vi "cluster.vi"() -> ()   [LabVIEW 2021]
panel:
  out "Array 2":T1(array[cluster])
  in  "y":enum16{"O", "B-", "B+", "A-", "A+"}(ring)
  out "Application form":T2
  in  "Array":T1(array[cluster])
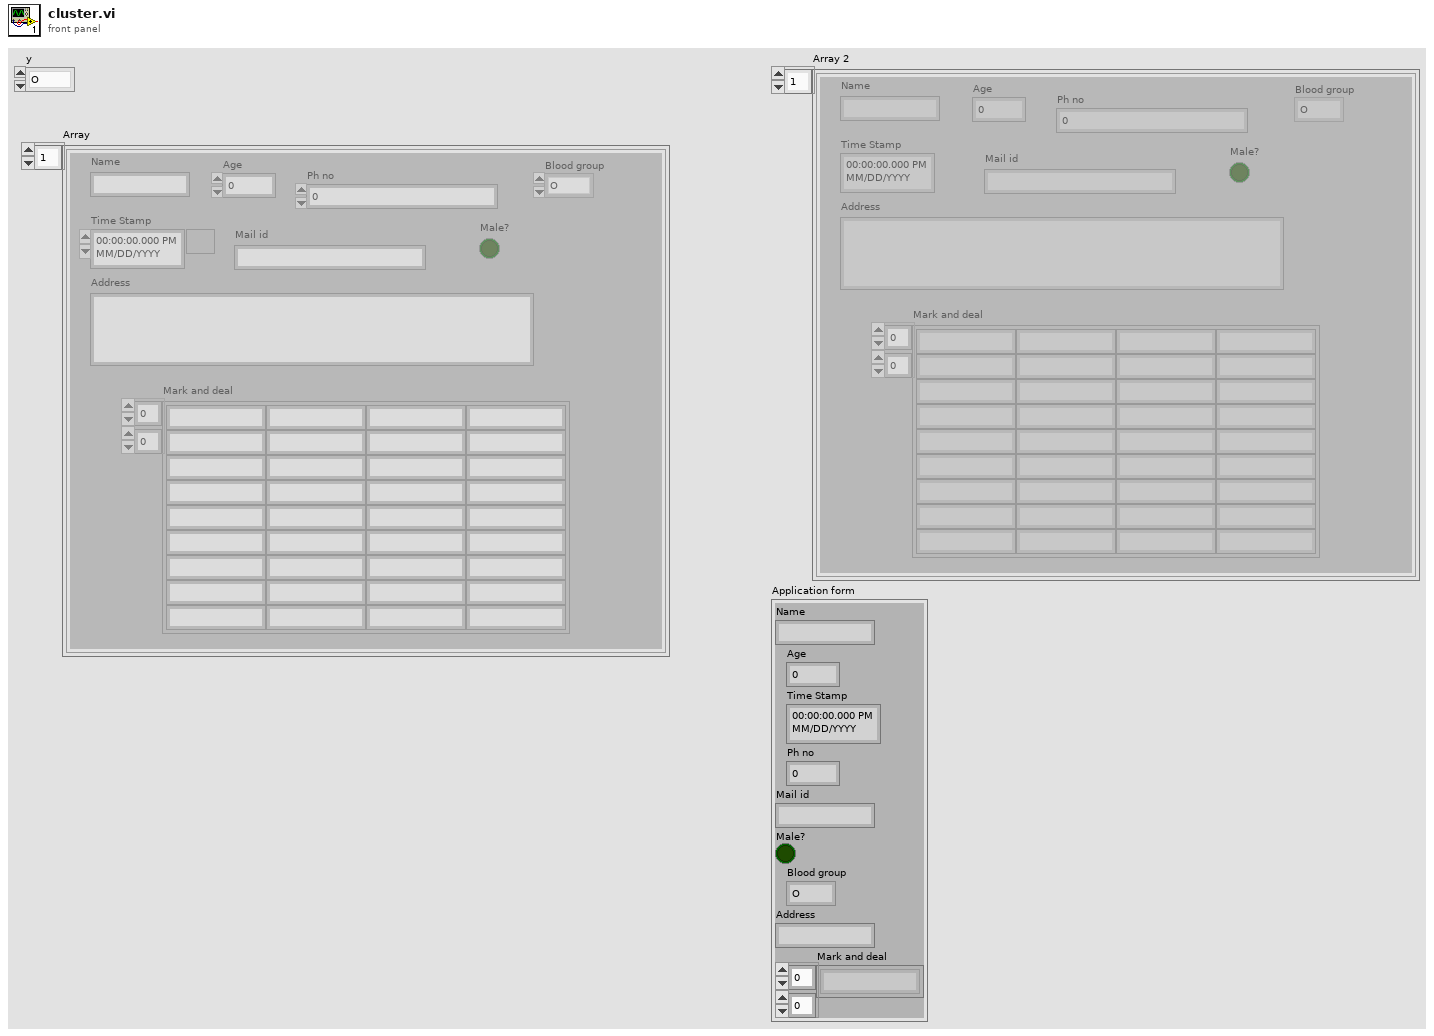
[diagram p1: front panel]
types:
  T1 = cluster{"Name":string, "Age":dbl, "Time Stamp":timestamp, "Ph no":dbl, "Mail id":string, "Male?":bool, "Blood group":enum16{"O", "B-", "B+", "A-", "A+"}, "Address":string, "Mark and deal":string[][]}[]
  T2 = cluster{"Name":string, "Age":dbl, "Time Stamp":timestamp, "Ph no":dbl, "Mail id":string, "Male?":bool, "Blood group":enum16{"O", "B-", "B+", "A-", "A+"}, "Address":string, "Mark and deal":string[][]}
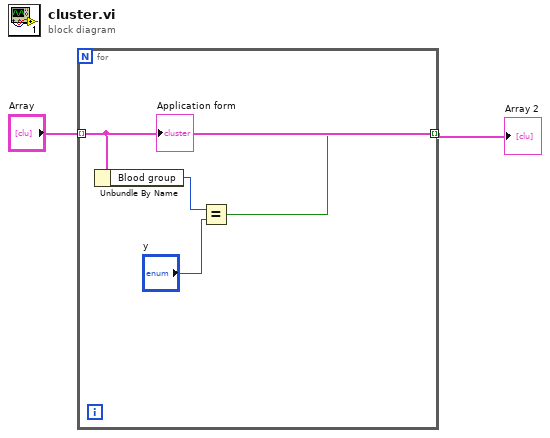
[diagram p0: block diagram]
diagram:
  n1 = for {
    tunnel: "Array" -> [w5] mode=indexing
    tunnel: "Array" -> [w2] mode=indexing
    n2 = Unbundle By Name(w5) -> ("Blood group"=w4:enum16{"O", "B-", "B+", "A-", "A+"})
    n3 = Equal?(x=w4, y="y") -> (x = y?=w2:bool)
    "Application form" <- w5
  }
  "Array 2" <- "Array"
